vi "Cluster to Array (recursive).vi"(8 "error in (no error)":errorcluster, 11 "Variant":variant) -> (0 "error out":errorcluster, 2 "Elements":variant[](array[variant]), 3 "Types":T1(array[ring]))   [LabVIEW 2013, in "PQ Connection.lvclass"]
uses:
  PQ Connection.lvclass
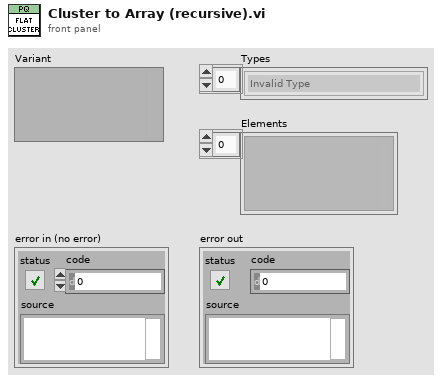
[diagram p1: front panel]
types:
  T1 = enum8{"Invalid Type", "Void", "I8", "I16", "I32", "I64", "U8", "U16", "U32", "U64", "Single Float", "Double Float", "Extended Float", "Single Complex", "Double Complex", "Extended Complex", "Enum U8", "Enum U16", "Enum U32", "Enum U64", "Single Float With Unit", "Double Float With Unit", "Extended Float With Unit", "Single Complex with Unit", "Double Complex with Unit", "Extended Complex with Unit", "Boolean", "String", "Path", "Picture", "Tag", "Array", "Cluster", "Variant", "LV Variant", "Waveform", "Timestamp", "Digital Waveform", "Digital Data", "ExpressData", "Refnum", "External Data", "VI", "Poly VI", "LabVIEW Class Instance", "Fixed Point"}[]
  T2 = typedef "Type Descriptor Enumeration__ogtk.ctl" = enum8{"<Null>", "I8", "I16", "I32", "I64", "U8", "U16", "U32", "U64", "SGL", "DBL", "EXT", "CSG", "CDB", "CXT", "0x0F", "0x10", "0x11", "0x12", "0x13", "0x14", "Enum U8", "Enum U16", "Enum U32", "Enum U64", "SGL PQ", "DBL PQ", "EXT PQ", "CSG PQ", "CDB PQ", "CXT PQ", "0x1F", "0x20", "Boolean", "0x22", "0x23", "0x24", "0x25", "0x26", "0x27", "0x28", "0x29", "0x2A", "0x2B", "0x2C", "0x2D", "0x2E", "0x2F", "String", "0x31", "Path", "Pict", "0x34", "0x35", "0x36", "DAQ", "0x38", "0x39", "0x3A", "0x3B", "0x3C", "0x3D", "0x3E", "0x3F", "Array", "0x41", "0x42", "0x43", "0x44", "0x45", "0x46", "0x47", "0x48", "0x49", "0x4A", "0x4B", "0x4C", "0x4D", "0x4E", "0x4F", "Cluster", "0x51", "0x52", "Variant", "Waveform", "0x55", "0x56", "0x57", "0x58", "0x59", "0x5A", "0x5B", "0x5C", "0x5D", "0x5E", "0x5F", "0x60", "0x61", "0x62", "0x63", "0x64", "0x65", "0x66", "0x67", "0x68", "0x69", "0x6A", "0x6B", "0x6C", "0x6D", "0x6E", "0x6F", "Refnum"}
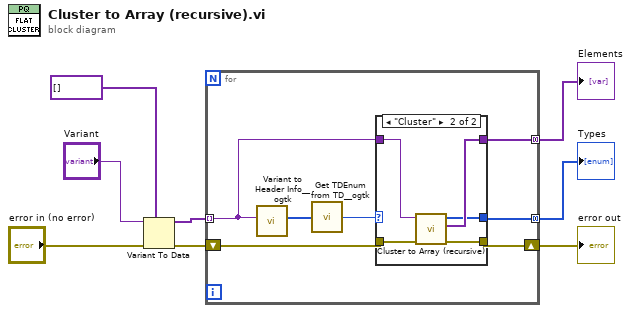
[diagram p0: block diagram]
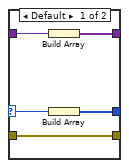
[diagram p2: hidden frame]
diagram:
  n1 = Variant To Data(error in="error in (no error)", type=variant[] [], Variant="Variant") -> (data=w6:variant[], error out=w2:errorcluster)
  n2 = for {
    tunnel: w6 -> [w11] mode=indexing
    tunnel: [w15] -> w7 mode=concatenating
    tunnel: [w14] -> w8 mode=concatenating
    shift-right: [w13] -> w1
    shift-left: w2 -> [w9]
    n3 = call "Variant to Header Info__ogtk.vi"("Variant"=w11) -> ("Type Descriptor"=w12:i16[])  [unwired: 3 in, 2 out]
    n4 = call <userlib>:"Get TDEnum from TD__ogtk.vi"("Type Descriptor"=w12) -> ("Type Descriptor Enumeration"=w10:T2)  [unwired: 4 in]
    n5 = case shown="\"Cluster\"" w10 {
      selector: w10 -> [w18 _]
      tunnel: w11 -> [w20 w25]
      tunnel: [w19 w24] -> w15
      tunnel: [w17 w23] -> w14
      tunnel: w9 -> [w16 w22]
      tunnel: [w16 w21] -> w13
      frame Default {
        n6 = Build Array(w20) -> (w19:variant[])
        n7 = Build Array(w18) -> (w17:T2[])
      }
      frame "Cluster" {
        n8 = call "Cluster to Array (recursive).vi"("error in (no error)"=w22, "Variant"=w25) -> ("error out"=w21:errorcluster, "Elements"=w24:variant[], "Types"=w23:T1)  [unwired: 7 in]
      }
    }
  }
  "Types" <- w8
  "Elements" <- w7
  "error out" <- w1
